vi "Mag calib panel.vi"(6 "Connection Status":T1={"MAC Address"="", "cnx handle"=0, "cnx flags"=0, "Address Type"=125, "Connection Interval (ms)"=125, "Timeout(ms)"=125, "Latency"=0, "bonding handle"=0} {"Address Type" items=["Public", "Random"]}, 8 "Error In":errorcluster, 11 "VISA resource in":refnum<visa-resource-name>) -> (0 "Error Out":errorcluster, 3 "VISA resource out":refnum<visa-resource-name>)   [LabVIEW 2016]
uses:
  <vilib>/Math Plots/3D Math Plots/3D Scatter/3D Scatter XCtrl/3D Scatter.xctl
  <vilib>/BLE/type_def/connection_status_bundle.ctl
  <vilib>/BLE/type_def/address_type.ctl
  Typedef/Mag calib - States.ctl
  Typedef/BLE char handle.ctl
  <vilib>/Math Plots/3D Math Plots/3D Scatter/3D Scatter Datatype/Public/Plot Helper (Vector).vi
  <vilib>/BLE/ble_functions/ble_write_by_handle_uint8array.vi
  <vilib>/Math Plots/3D Math Plots/3D Scatter/3D Scatter Datatype/3D Scatter Datatype.lvclass
panel:
  in  "Set & Save":bool
  in  "Exit":bool
  in  "Next":bool
  out "Calibration results":i32(listbox)
  out "Instructions":string="Press START CALIBRATION to begin magnetometer calibration"
  out "3D Mag Scatter":refnum<class "3D Plot Datatype.lvclass">[](xcontrol)
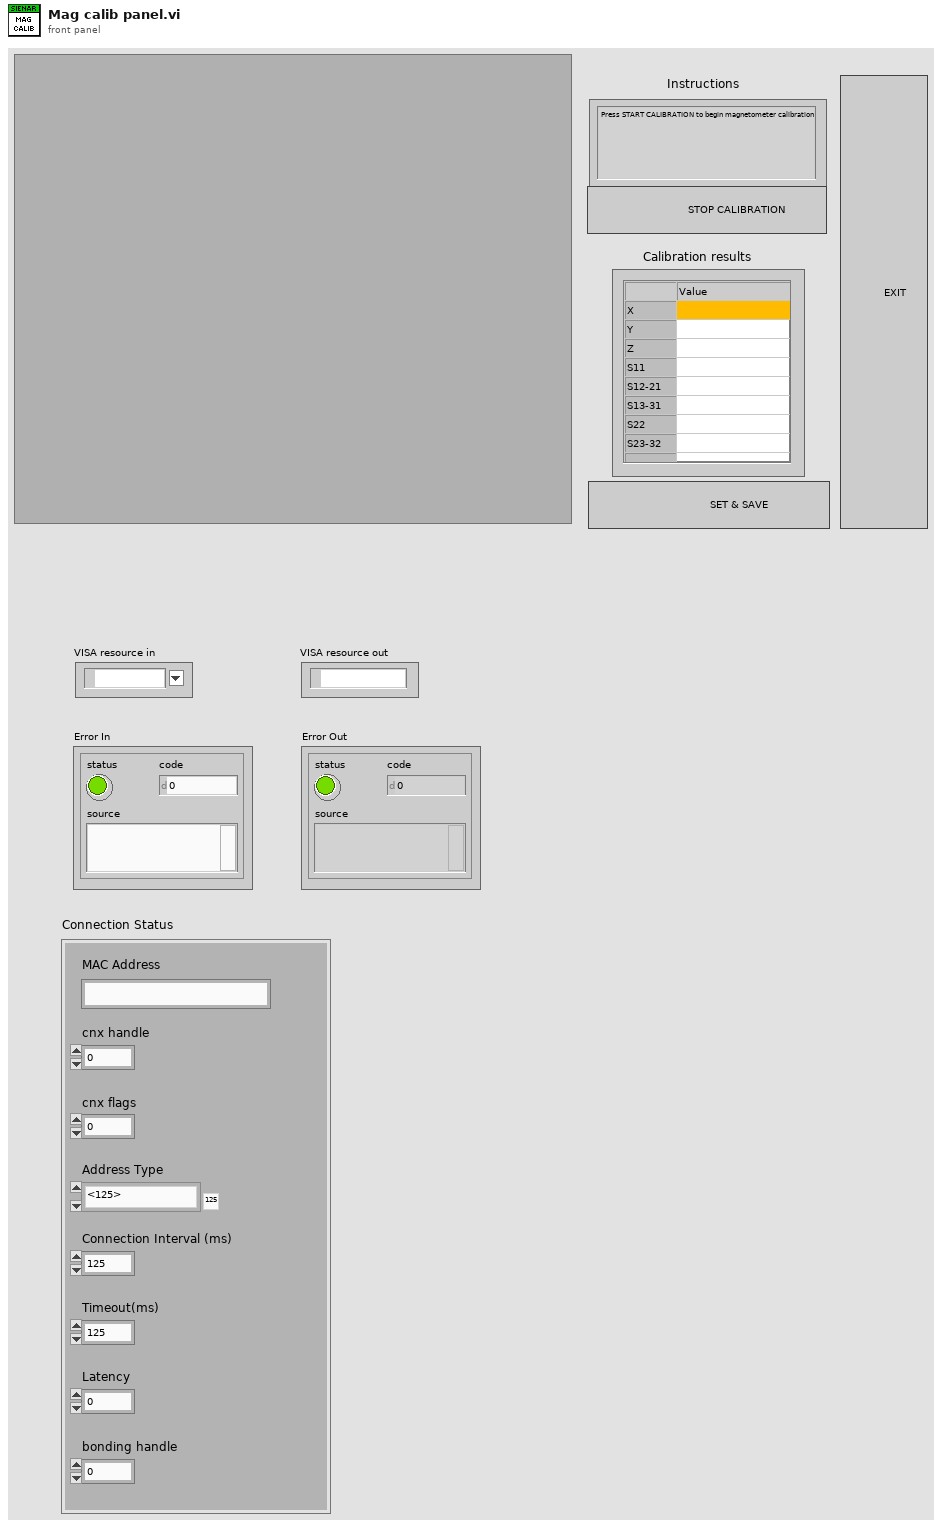
[diagram p1: front panel]
types:
  T1 = typedef "connection_status_bundle.ctl" = cluster{"MAC Address":string, "cnx handle":u8, "cnx flags":u8, "Address Type":T2, "Connection Interval (ms)":u16, "Timeout(ms)":u16, "Latency":u16, "bonding handle":u8}
  T2 = typedef "address_type.ctl" = u8
  T3 = cluster{"OffsetX":i16, "OffsetY":i16, "OffsetZ":i16, "A11":sgl, " A12":sgl, "A13":sgl, "A22":sgl, "A23":sgl, "A33":sgl}
  T4 = typedef "Mag calib - States.ctl" = enum16{"Start calibration", "Acquire Mag data", "Plot data", "Calibrate data", "Set & Save", "Exit"}
  T5 = enum16{"Accelerometer", "Gyroscope", "Magnetometer"}
  T6 = typedef "BLE char handle.ctl" = u16
  T7 = cluster{"AccelData":cluster{"AccelX":i16, "AccelY":i16, "AccelZ":i16}, "GyroData":cluster{"GyroX":i16, "GyroY":i16, "GyroZ":i16}, "MagData":cluster{"MagX":i16, "MagY":i16, "MagZ":i16}}
  T8 = cluster{"AccelData":cluster{"AccelX":dbl, "AccelY":dbl, "AccelZ":dbl}, "GyroData":cluster{"GyroX":dbl, "GyroY":dbl, "GyroZ":dbl}, "MagData":cluster{"MagX":dbl, "MagY":dbl, "MagZ":dbl}}
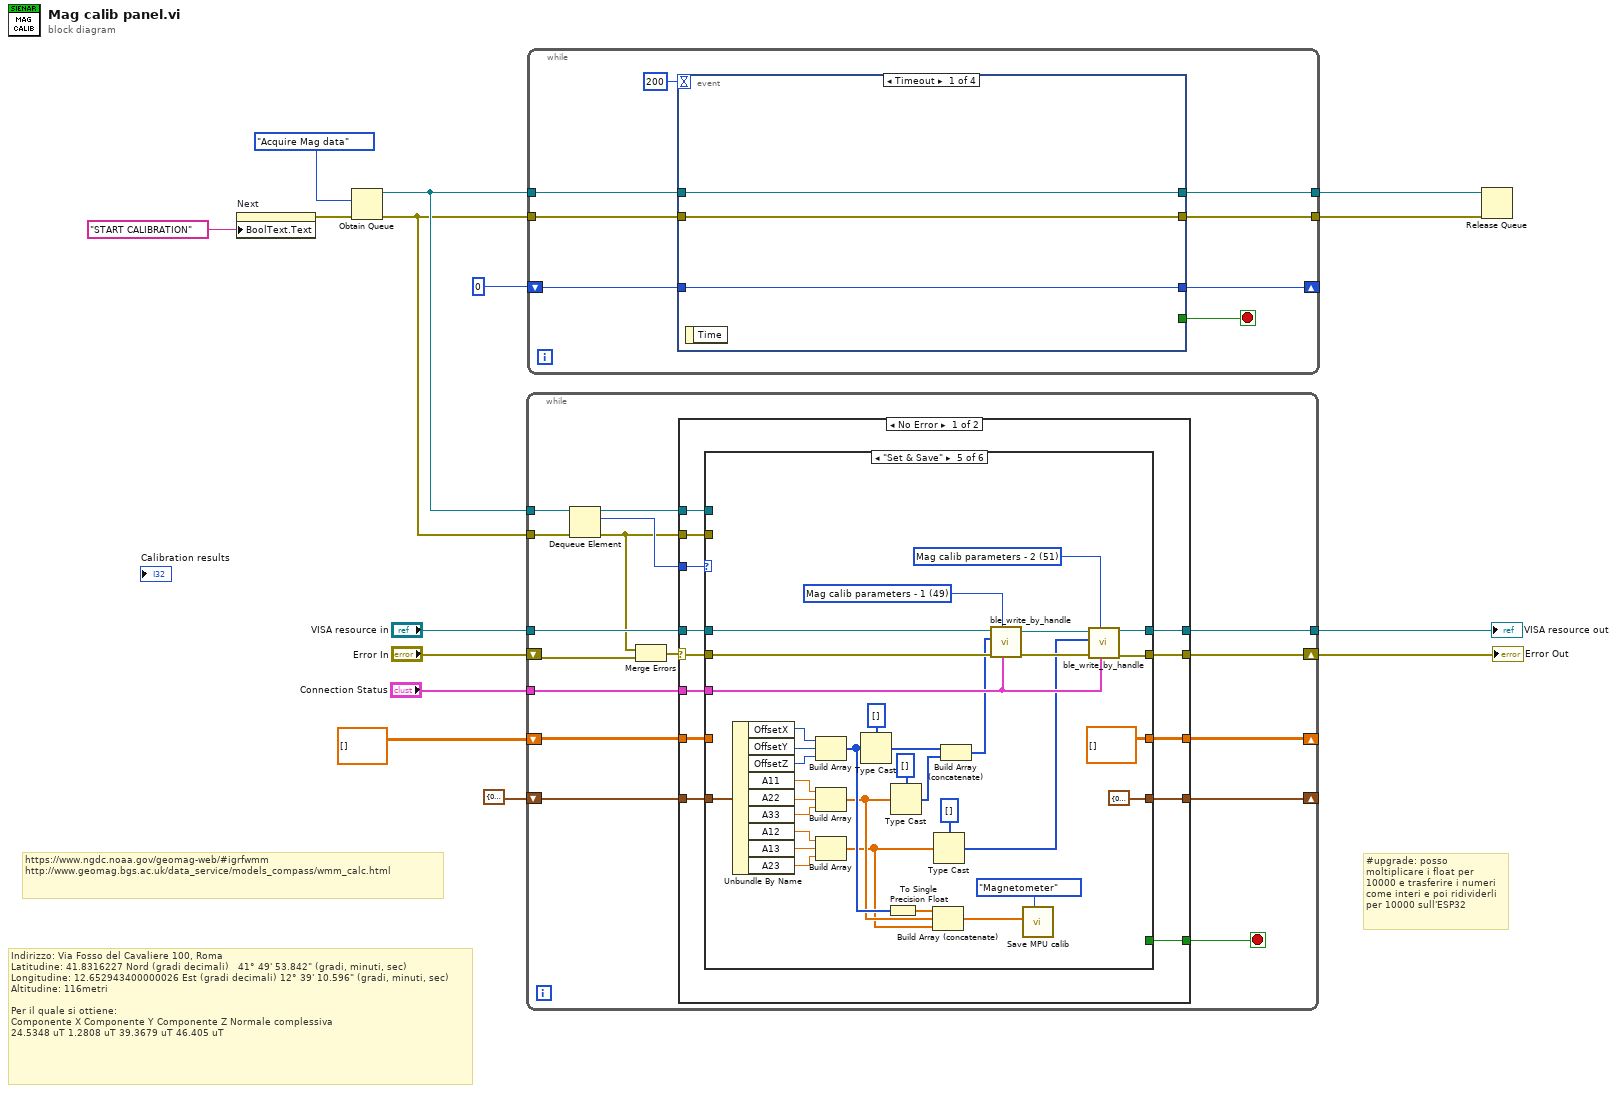
[diagram p0: block diagram]
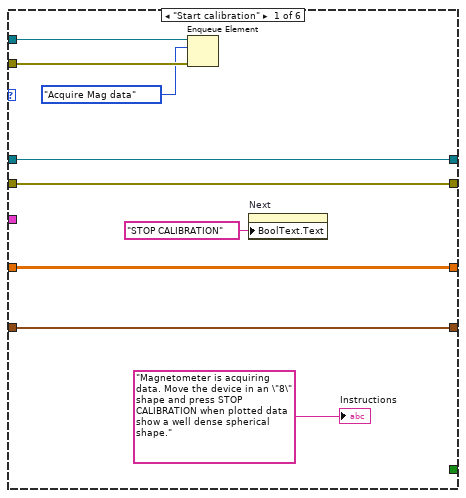
[diagram p2: hidden frame]
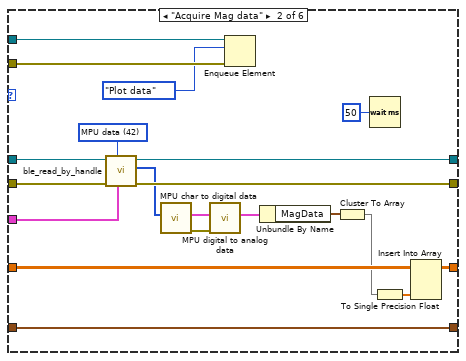
[diagram p3: hidden frame]
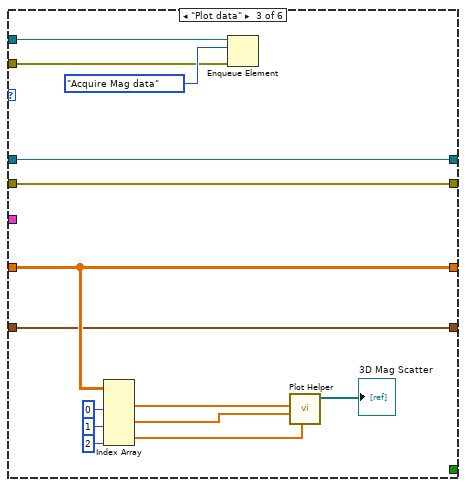
[diagram p4: hidden frame]
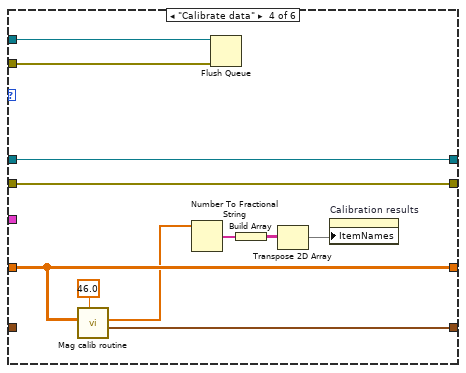
[diagram p5: hidden frame]
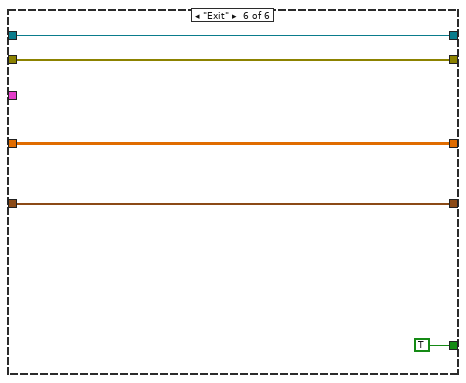
[diagram p6: hidden frame]
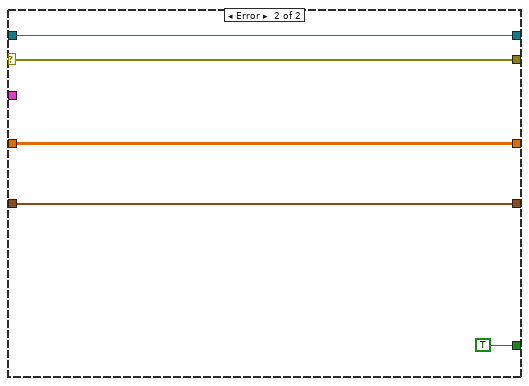
[diagram p7: hidden frame]
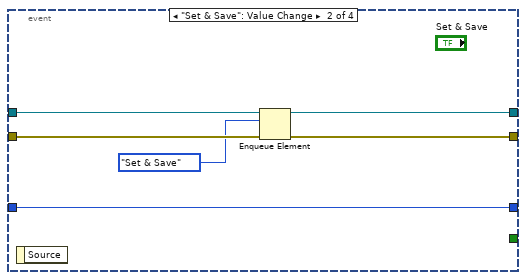
[diagram p8: hidden frame]
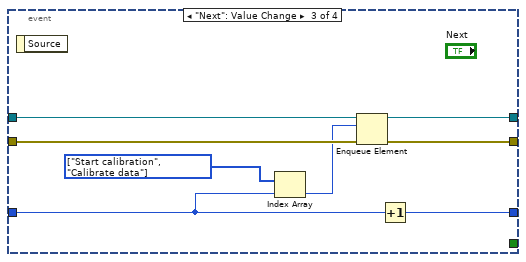
[diagram p9: hidden frame]
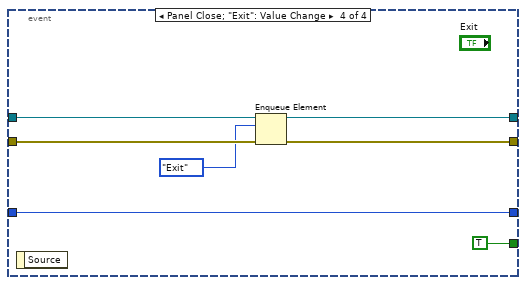
[diagram p10: hidden frame]
diagram:
  # "#upgrade: posso\nmoltiplicare i float per\n10000 e trasferire i numeri\ncome interi e poi ridividerli\nper 10000 sull'ESP32"
  # "Indirizzo: Via Fosso del Cavaliere 100, Roma\nLatitudine: 41.8316227 Nord (gradi decimali) \t\t41° 49' 53.842\" (gradi, minuti, sec)\nLongitudine: 12.652943400000026 Est (gradi decimali)\t12° 39' 10.596\" (gradi, minuti, sec)\nAltitudine: 116metri\n\nPer il quale si ottiene:\nComponente X\tComponente Y\tComponente Z\tNormale complessiva\n24.5348 uT\t1.2808 uT\t39.3679 uT\t46.405 uT"
  # "https://www.ngdc.noaa.gov/geomag-web/#igrfwmm\nhttp://www.geomag.bgs.ac.uk/data_service/models_compass/wmm_calc.html"
  n1 = property on="Next" class="Bool"("BoolText.Text"="START CALIBRATION" ("Boolean Text.Text")) -> (error out=w3:errorcluster)  [unwired: 2 in, 1 out]
  n2 = Obtain Queue(element data type=Mag_calib_-_States."Acquire Mag data", error in (no error)=w3) -> (queue out=w15:refnum<queue>, error out=w14:errorcluster)  [unwired: 3 in, 1 out]
  n3 = while {
    tunnel: w15 -> [w31]
    tunnel: w14 -> [w30]
    shift-right: [w25] -> w6
    shift-left: "Error In" -> [w19]
    tunnel: "VISA resource in" -> [w27]
    tunnel: [w26] -> w7
    tunnel: "Connection Status" -> [w24]
    shift-right: [w21] -> _
    shift-left: sgl[][] [] ("Uncalibrated data") -> [w23]
    shift-right: [w16] -> _
    shift-left: T3 {"OffsetX"=0, "OffsetY"=0, "OffsetZ"=0, "A11"=0.0, " A12"=0.0, "A13"=0.0, "A22"=0.0, "A23"=0.0, "A33"=0.0} ("Calib data") -> [w20]
    stop <- w22 stop-if-true
    n4 = Dequeue Element(queue=w31, error in (no error)=w30) -> (queue out=w28:refnum<queue>, element=w29:T4, error out=w18:errorcluster)  [unwired: 1 in, 1 out]
    n5 = Merge Errors(w18, w19) -> (w17:errorcluster)
    n6 = case shown="No Error" w17 {
      selector: w17 -> [w33 w141]
      tunnel: w29 -> [w44 _]
      tunnel: w28 -> [w43 _]
      tunnel: w18 -> [w42 _]
      tunnel: w27 -> [w41 w142]
      tunnel: [w40 w142] -> w26
      tunnel: [w39 w141] -> w25
      tunnel: w24 -> [w38 _]
      tunnel: w23 -> [w37 w140]
      tunnel: [w36 TRUE] -> w22
      tunnel: [w35 w140] -> w21
      tunnel: w20 -> [w34 w138]
      tunnel: [w32 w138] -> w16
      frame No Error {
        n7 = case shown="\"Set & Save\"" w44 {
          tunnel: w43 -> [w50 w73 w76 w93 _ _]
          tunnel: w42 -> [w49 w72 w75 w92 _ _]
          tunnel: w41 -> [w53 w70 w86 w98 w129 w136]
          tunnel: w33 -> [w52 w69 w85 w97 w130 w135]
          tunnel: [w53 w68 w86 w98 w128 w136] -> w40
          tunnel: [w52 w67 w85 w97 w127 w135] -> w39
          tunnel: w38 -> [_ w66 _ _ w126 _]
          tunnel: w37 -> [w51 w58 w84 w95 _ w134]
          tunnel: [_ _ _ _ _ TRUE] -> w36
          tunnel: [w51 w59 w84 w95 sgl[][] [] ("Uncalibrated data") w134] -> w35
          tunnel: w34 -> [w45 w55 w74 _ w117 w133]
          tunnel: [w45 w55 w74 w88 T3 {"OffsetX"=0, "OffsetY"=0, "OffsetZ"=0, "A11"=0.0, " A12"=0.0, "A13"=0.0, "A22"=0.0, "A23"=0.0, "A33"=0.0} ("Calib data") w133] -> w32
          frame "Start calibration" {
            n8 = Enqueue Element(queue=w50, element=Mag_calib_-_States."Acquire Mag data", error in (no error)=w49) -> ()  [unwired: 1 in, 3 out]
            n9 = property on="Next" class="Bool"("BoolText.Text"="STOP CALIBRATION" ("Boolean Text.Text")) -> ()  [unwired: 2 in, 2 out]
            "Instructions" <- "Magnetometer is acquiring data. Move the device in an \"8\" shape and press STOP CALIBRATION when plotted data show a well dense spherical shape."
          }
          frame "Acquire Mag data" {
            w54 = T6 42 items=["MPU data"=42, "MPU data - DESCR"=43, "Accel calib parameters"=45, "Gyro calib parameters"=47, "Mag calib parameters - 1"=49, "Mag calib parameters - 2"=51, "YPR"=53, "YPR - DESCR"=54, "Strain sensors"=56, "Strain sensors - DESCR"=57, "Wristband"=59, "Wristband - DESCR"=60] ("BLE char handle")
            n10 = call <vilib>:"ble_read_by_handle.vi"("Connection Status"=w66, "Handle"=w54, "error in (no error)"=w69, "COM Bluegiga in"=w70) -> ("error out"=w67:errorcluster, "characteristic value"=w65:u8[], "COM Bluegiga out"=w68:refnum<visa-resource-name>)  [unwired: 5 in]
            n11 = call "MPU char to digital data.vi"("MPU characteristic data"=w65) -> ("Error Out"=w63:errorcluster, "Digital MPU data"=w62:T7)  [unwired: 9 in]
            n12 = call "MPU digital to analog data.vi"("Error In"=w63, "Digital MPU data"=w62) -> ("Analog MPU data"=w61:T8)  [unwired: 8 in, 1 out]
            n13 = Enqueue Element(queue=w73, element=Mag_calib_-_States."Plot data", error in (no error)=w72) -> ()  [unwired: 1 in, 3 out]
            n14 = Unbundle By Name(w61) -> ("MagData"=w60:cluster{"MagX":dbl, "MagY":dbl, "MagZ":dbl})
            n15 = Cluster To Array(cluster=w60) -> (array=w57:dbl[])
            n16 = Wait (ms)(milliseconds to wait=u32 50) -> ()  [unwired: 1 out]
            n17 = To Single Precision Float(number=w57) -> (single precision float=w56:sgl[])
            n18 = Insert Into Array(array=w58, new element=w56) -> (w59:sgl[][])  [unwired: 2 in]
          }
          frame "Plot data" {
            n19 = Index Array(array=w84, index (col) #1=0 ("disabled index (col)"), index (col) #2=1 ("index (col)"), index (col) #3=2 ("index (col)")) -> (element #1=w80:sgl[], element #2=w79:sgl[], element #3=w78:sgl[])  [unwired: 3 in]
            n20 = Enqueue Element(queue=w76, element=Mag_calib_-_States."Acquire Mag data", error in (no error)=w75) -> ()  [unwired: 1 in, 3 out]
            n21 = call-poly <vilib>:"Plot Helper.vi"("z vector"=w78, "y vector"=w79, "x vector"=w80) -> ("3D Plot lvclass Array out"=→"3D Mag Scatter":refnum<class "3D Plot Datatype.lvclass">[])  [unwired: 3 in, 5 out]
          }
          frame "Calibrate data" {
            n22 = call "Mag calib routine.vi"("Norm field"=46.0, "Uncalibrated data"=w95) -> (1:"Calib data"=w88:T3, 2:"Calib data"=w91:sgl[])  [unwired: 6 in, 2 out]
            n23 = Number To Fractional String(number=w91) -> (F-format string=w94:string[])  [unwired: 3 in]
            n24 = Flush Queue(queue=w93, error in (no error)=w92) -> ()  [unwired: 3 out]
            n25 = Build Array(w94) -> (w90:string[][])
            n26 = Transpose 2D Array(2D array=w90) -> (transposed array=w89:string[][])
            n27 = property on="Calibration results" class="MCListbox (strict)"("ItemNames"=w89) -> ()  [unwired: 2 in, 2 out]
          }
          frame "Set & Save" {
            w99 = T6 51 items=["MPU data"=42, "MPU data - DESCR"=43, "Accel calib parameters"=45, "Gyro calib parameters"=47, "Mag calib parameters - 1"=49, "Mag calib parameters - 2"=51, "YPR"=53, "YPR - DESCR"=54, "Strain sensors"=56, "Strain sensors - DESCR"=57, "Wristband"=59, "Wristband - DESCR"=60] ("BLE char handle")
            w100 = T6 49 items=["MPU data"=42, "MPU data - DESCR"=43, "Accel calib parameters"=45, "Gyro calib parameters"=47, "Mag calib parameters - 1"=49, "Mag calib parameters - 2"=51, "YPR"=53, "YPR - DESCR"=54, "Strain sensors"=56, "Strain sensors - DESCR"=57, "Wristband"=59, "Wristband - DESCR"=60] ("BLE char handle")
            n28 = Unbundle By Name(w117) -> ("OffsetX"=w116:i16, "OffsetY"=w115:i16, "OffsetZ"=w114:i16, "A11"=w112:sgl, "A22"=w113:sgl, "A33"=w111:sgl, "A12"=w109:sgl, "A13"=w110:sgl, "A23"=w108:sgl)
            n29 = Build Array(w116, w115, w114) -> (w106:i16[])
            n30 = Build Array(w112, w113, w111) -> (w104:sgl[])
            n31 = Build Array(w109, w110, w108) -> (w103:sgl[])
            n32 = Type Cast(type=u8[] [], x=w106) -> (*(type *) &x=w121:u8[])
            n33 = To Single Precision Float(number=w106) -> (single precision float=w105:sgl[])
            n34 = Type Cast(type=u8[] [], x=w104) -> (*(type *) &x=w122:u8[])
            n35 = Build Array (concatenate)(w105, w104, w103) -> (w102:sgl[])
            n36 = Type Cast(type=u8[] [], x=w103) -> (*(type *) &x=w119:u8[])
            n37 = Build Array (concatenate)(w121, w122) -> (w120:u8[])
            n38 = call-poly <vilib>:"ble_write_by_handle.vi"("Connection Status"=w126, "Handle"=w100, "error in (no error)"=w130, "data (uint8array)"=w120, "COM Bluegiga in"=w129) -> ("error out"=w125:errorcluster, "COM Bluegiga out"=w124:refnum<visa-resource-name>)  [unwired: 5 in]
            n39 = call "Save MPU calib.vi"("Calib data type"=T5."Magnetometer", "Calib data"=w102) -> ()  [unwired: 9 in, 1 out]
            n40 = call-poly <vilib>:"ble_write_by_handle.vi"("Connection Status"=w126, "Handle"=w99, "error in (no error)"=w125, "data (uint8array)"=w119, "COM Bluegiga in"=w124) -> ("error out"=w127:errorcluster, "COM Bluegiga out"=w128:refnum<visa-resource-name>)  [unwired: 5 in]
          }
          frame "Exit" {
          }
        }
      }
      frame Error {
      }
    }
  }
  "VISA resource out" <- w7
  "Error Out" <- w6
  n41 = while {
    tunnel: w15 -> [w150]
    tunnel: w14 -> [w149]
    tunnel: [w148] -> w12
    tunnel: [w147] -> w11
    shift-right: [w143] -> _
    shift-left: 0 -> [w144]
    stop <- w145 stop-if-true
    n42 = event shown="[0] Timeout" {
      selector: _ -> [_ _ _ _]
      dyn-events: _ -> [_ _ _ _]
      timeout: 200 -> [_ _ _ _]
      tunnel: w150 -> [w153 w159 w167 w174]
      tunnel: w149 -> [w152 w158 w166 w172]
      tunnel: [w153 w157 w165 w173] -> w148
      tunnel: [w152 w156 w164 w171] -> w147
      tunnel: [_ _ _ TRUE] -> w145
      tunnel: w144 -> [w151 w154 w163 w168]
      tunnel: [w151 w154 w162 w168] -> w143
      event Timeout {
        n43 = event-data() -> ()  [unwired: 1 in, 1 out]
      }
      event "Set & Save": Value Change {
        n44 = event-data() -> ()  [unwired: 1 in, 1 out]
        n45 = Enqueue Element(queue=w159, element=Mag_calib_-_States."Set & Save", error in (no error)=w158) -> (queue out=w157:refnum<queue>, error out=w156:errorcluster)  [unwired: 1 in, 1 out]
      }
      event "Next": Value Change {
        w161 = T4[] [enum."Start calibration", enum."Calibrate data"] items=["Start calibration", "Acquire Mag data", "Plot data", "Calibrate data", "Set & Save", "Exit"]
        n46 = event-data() -> ()  [unwired: 1 in, 1 out]
        n47 = Index Array(array=w161, index=w163) -> (element=w160:T4)
        n48 = Enqueue Element(queue=w167, element=w160, error in (no error)=w166) -> (queue out=w165:refnum<queue>, error out=w164:errorcluster)  [unwired: 1 in, 1 out]
        n49 = Increment(x=w163) -> (x+1=w162:i32)
      }
      event Panel Close; "Exit": Value Change {
        n50 = event-data() -> ()  [unwired: 1 in, 1 out]
        n51 = Enqueue Element(queue=w174, element=Mag_calib_-_States."Exit", error in (no error)=w172) -> (queue out=w173:refnum<queue>, error out=w171:errorcluster)  [unwired: 1 in, 1 out]
      }
    }
  }
  n52 = Release Queue(queue=w12, error in (no error)=w11) -> ()  [unwired: 1 in, 3 out]
